vi "Main - Add Local Chassis.vi"(8 "error in (no error)":errorcluster, 11 "Node Ptr":u64 format="%.0x") -> (0 "error out":errorcluster)   [LabVIEW 2016, in "Scan Engine Custom Device.lvlib"]
uses:
  Scan Engine Custom Device.lvlib
  <vilib>/NI Veristand/Custom Device API/Custom Device API.lvlib
  Globals/Scan Engine GUIDs.vi
  Globals/Property Strings.vi
  Type Defs/Host - FPGAScanInterfaceMode.ctl
panel:
  in  "Tag":string
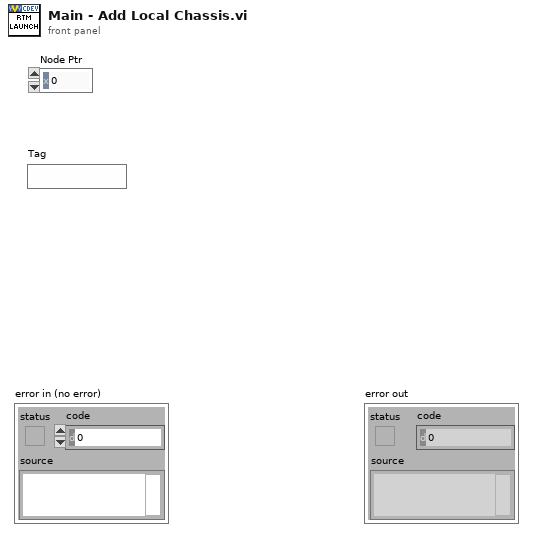
[diagram p1: front panel]
types:
  T1 = typedef "Scan Engine Custom Device.lvlib/Host - FPGAScanInterfaceMode.ctl" = enum16{"Use Current", "FPGA", "Scan Mode"}
  T2 = typedef "Custom Device API.lvlib/Custom Device Item Ref.ctl" = u64
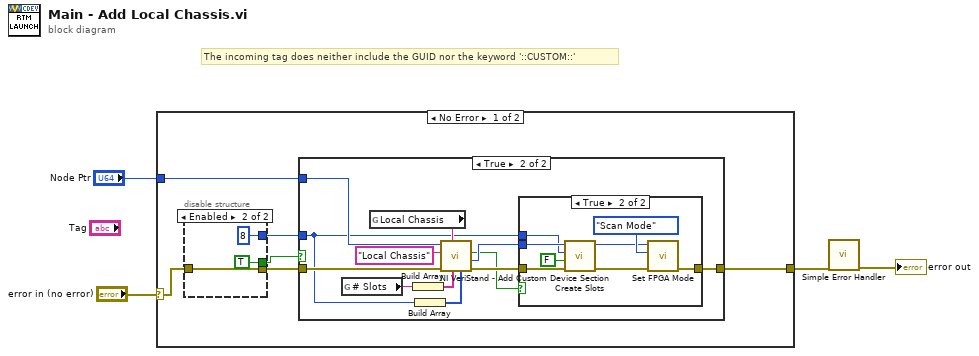
[diagram p0: block diagram]
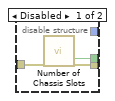
[diagram p2: hidden frame]
diagram:
  # "The incoming tag does neither include the GUID nor the keyword '::CUSTOM::'"
  n1 = case shown="No Error" "error in (no error)" {
    selector: "error in (no error)" -> [w5 w39]
    tunnel: "Node Ptr" -> [w7 _]
    tunnel: [w6 w39] -> w2
    frame No Error {
      n2 = disable-structure shown="Enabled" {
        disable-tunnel: [_ 8 ("# Slots")] -> w10
        disable-tunnel: [w13 w14] -> w9
        disable-tunnel: [w12 TRUE ("OK")] -> w8
        disable-tunnel: w5 -> [w11 w14]
        frame Disabled {
          n3 = call "Number of Chassis Slots"("error in (no error)"=w11) -> ("OK"=w12:bool, "error out"=w13:errorcluster)  [unwired: 16 in, 1 out]
        }
        frame Enabled {
        }
      }
      n4 = case shown="True" w8 {
        tunnel: w10 -> [_ w21]
        tunnel: w7 -> [_ w25]
        tunnel: w9 -> [w17 w24]
        tunnel: [w17 w19] -> w6
        frame False {
        }
        frame True {
          n5 = global read "Property Strings.vi" "# Slots"() -> (w22:string)
          n6 = global read "Scan Engine GUIDs.vi" "Local Chassis"() -> (w28:string)
          n7 = Build Array(w22) -> (w23:string[])
          n8 = Build Array(w21) -> (w20:i32[])
          n9 = call <vilib>:"NI VeriStand - Add Custom Device Section.vi"("Property Values"=w20, "Property names"=w23, "GUID (Default Section)"=w28, "error in (no error)"=w24, "Section Name"="Local Chassis", "Parent Ref in"=w25) -> ("error out"=w26:errorcluster, "Section Ptr"=w27:T2, "Newly Created?"=w18:bool)  [unwired: 2 in, 1 out]
          n10 = case shown="True" w18 {
            tunnel: w27 -> [_ w37]
            tunnel: w26 -> [w30 w36]
            tunnel: w21 -> [_ w35]
            tunnel: [w30 w33] -> w19
            frame False {
            }
            frame True {
              n11 = call "Create Slots.vi"("error in"=w36, "EtherCAT?"=FALSE, "Num Slots"=w35, "Item Ref In"=w37) -> ("error out"=w34:errorcluster, "Item Ref out"=w31:T2)  [unwired: 5 in]
              n12 = call "Set FPGA Mode.vi"("error in (no error)"=w34, "FPGAScanInterfaceMode"=Host_-_FPGAScanInterfaceMode."Scan Mode", "Item Ref in"=w31) -> ("error out"=w33:errorcluster)  [unwired: 7 in, 1 out]
            }
          }
        }
      }
    }
    frame Error {
    }
  }
  n13 = call <vilib>:"Simple Error Handler.vi"("error in (no error)"=w2) -> ("error out"=→"error out":errorcluster)  [unwired: 4 in, 4 out]
